vi "Read List Operation.vi"(8 "error in (no error)":errorcluster, 9 "List Step Number(0)":dbl, 10 "List Operation(0:Voltage)":u16(ring) items=["Voltage", "Current"], 11 "VISA resource name":refnum<visa-resource-name>) -> (0 "error out":errorcluster, 1 "List Operation":string, 2 "List Mode":string, 3 "VISA resource name out":refnum<visa-resource-name>)   [LabVIEW 2021, in "Keithley 2200 Series.lvlib"]
doc: "Reads the list operation mode and the list repeat mode."
uses:
  <instrlib>/Keithley 2200 Series/Keithley 2200 Series.lvlib
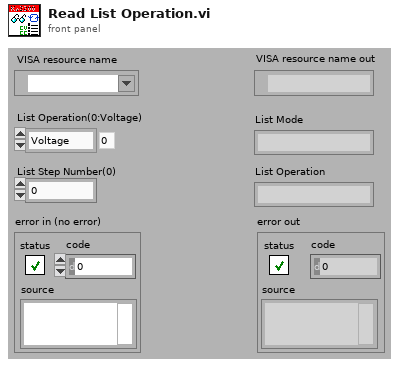
[diagram p1: front panel]
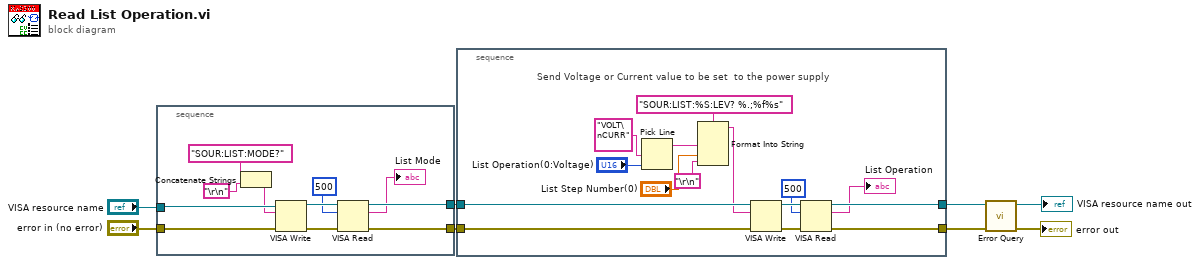
[diagram p0: block diagram]
diagram:
  n1 = stacked-sequence {
    tunnel: "error in (no error)" -> [w19]
    tunnel: "VISA resource name" -> [w18]
    tunnel: [w14] -> w6
    tunnel: [w13] -> w5
    frame #0 {
      n2 = Concatenate Strings("SOUR:LIST:MODE?" ("format string"), "\r\n") -> (w10:string)
      n3 = VISA Write(VISA resource name=w18, write buffer=w10, error in (no error)=w19) -> (VISA resource name out=w17:refnum<visa-resource-name>, error out=w16:errorcluster)  [unwired: 1 out]
      n4 = VISA Read(VISA resource name=w17, byte count=u32 500, error in (no error)=w16) -> (VISA resource name out=w14:refnum<visa-resource-name>, read buffer=→"List Mode":string, error out=w13:errorcluster)  [unwired: 1 out]
    }
  }
  n5 = stacked-sequence {
    tunnel: w6 -> [w30]
    tunnel: w5 -> [w29]
    tunnel: [w24] -> w4
    tunnel: [w23] -> w3
    frame #0 {
      # "Send Voltage or Current value to be set  to the power supply"
      n6 = Pick Line(multi-line string="VOLT\nCURR" ("format string"), line index="List Operation(0:Voltage)") -> (output string=w32:string)  [unwired: 1 out]
      n7 = Format Into String(format string="SOUR:LIST:%S:LEV? %.;%f%s", w32, "List Step Number(0)", "\r\n") -> (resulting string=w28:string)  [unwired: 2 in, 1 out]
      n8 = VISA Write(VISA resource name=w30, write buffer=w28, error in (no error)=w29) -> (VISA resource name out=w26:refnum<visa-resource-name>, error out=w27:errorcluster)  [unwired: 1 out]
      n9 = VISA Read(VISA resource name=w26, byte count=u32 500, error in (no error)=w27) -> (VISA resource name out=w24:refnum<visa-resource-name>, read buffer=→"List Operation":string, error out=w23:errorcluster)  [unwired: 1 out]
    }
  }
  n10 = call <instrlib>:"Error Query.vi"("error in (no error)"=w3, "VISA resource name"=w4) -> ("error out"=→"error out":errorcluster, "VISA resource name out"=→"VISA resource name out":refnum<visa-resource-name>)  [unwired: 8 out]
